vi "SeCrTs-DI SEQ MAIN.vi"(8 "error in":errorcluster, 11 "Message Queue":refnum<queue>) -> (0 "error Out":errorcluster)   [LabVIEW 2022 SP3]
uses:
  <vilib>/Platform/TimedLoop/XDataNode/timing_clust.ctl
  <vilib>/Platform/TimedLoop/XDataNode/nitl_modes.ctl
  <vilib>/Platform/TimedLoop/XDataNode/wakeup.ctl
  RT Controls/SeCrTs-FGV Read write.ctl
  <vilib>/platform/TimedLoop/XDataNode/XDataNode.xnode
  <vilib>/Platform/TimedLoop/XDataNode/XDNodeRunTimeDep.lvlib
panel:
  out "output array":string[](array[string])
  out "x-y":u32
  out "Numeric":i32
  out "Failure \ncase Seq":string[](array[string])
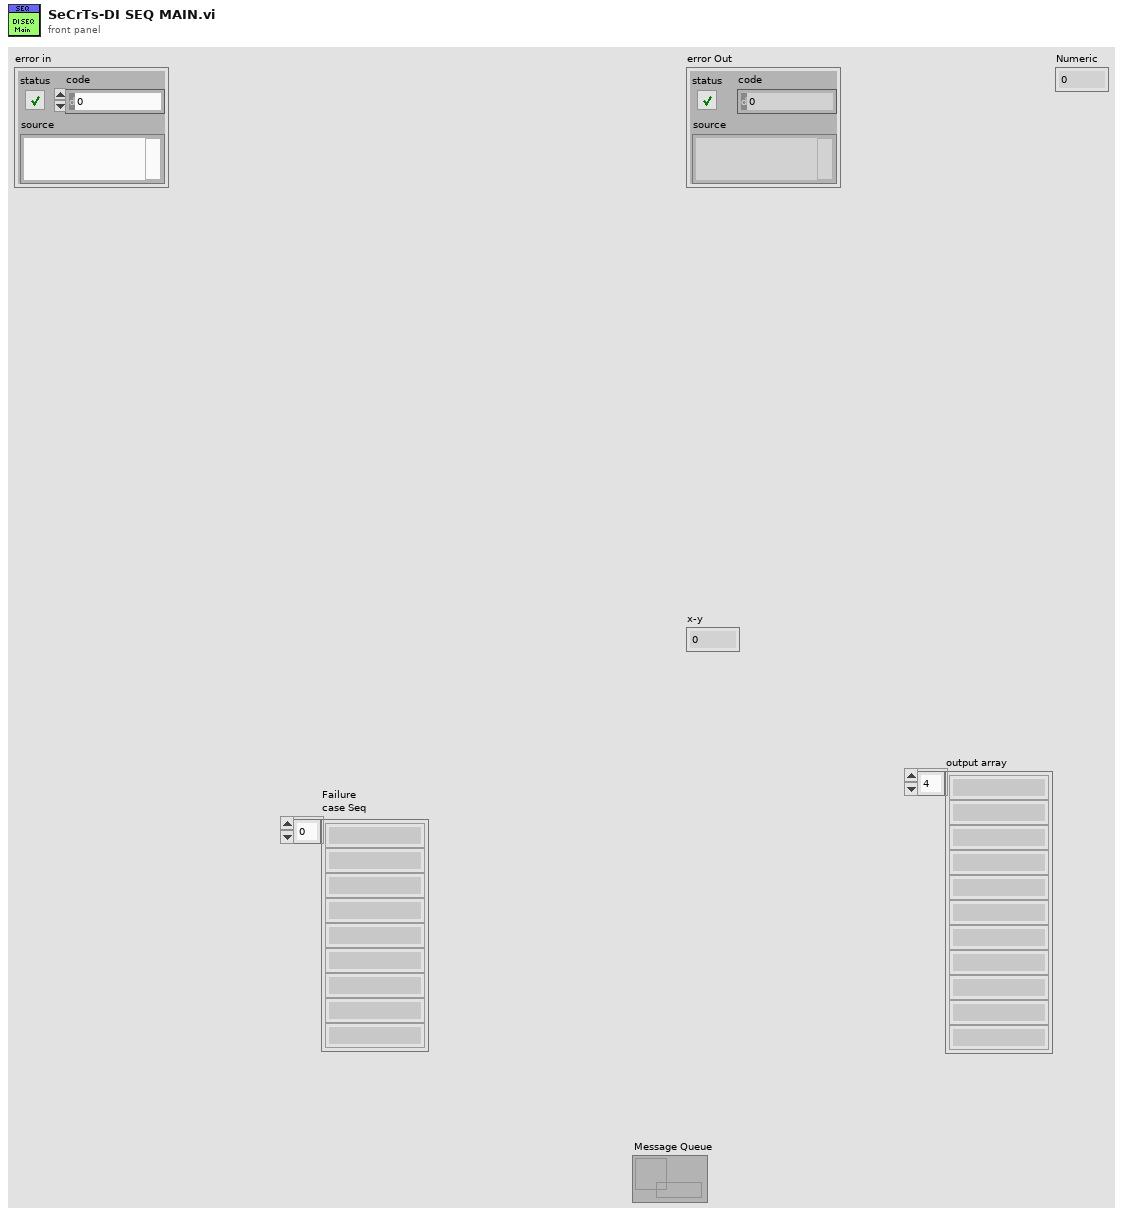
[diagram p1: front panel]
types:
  T1 = typedef "XDNodeRunTimeDep.lvlib/timing_clust.ctl" = cluster{"Expected End [f-1]":u64, "Actual End [f-1]":u64, "Finished Late? [f-1]":bool, "Expected End [i-1]":u64, "Actual End [i-1]":u64, "Finished Late? [i-1]":bool, "Expected Start [i]":u64, "Actual Start [i]":u64, "Expected Start [f]":u64, "Actual Start [f]":u64, "Source Name":string, "Structure Name":string, "Period":i64, "Deadline":i64, "Offset":i64, "Start":i64, "Priority":i32, "Timeout":i32, "Mode":T2, "Wakeup Reason":T3, "Error":errorcluster, "Source Type":string, "Secondary Source Type":string, "Global End Time":u64, "Global Start Time":u64, "Frame Duration":u64, "Iteration Duration":u64, "Assigned CPU":i32, "I/O Scan Engine Mode":u32}
  T2 = typedef "XDNodeRunTimeDep.lvlib/nitl_modes.ctl" = enum32{"No Change", "Process missed periods, maintain original phase", "Discard missed periods, maintain original phase", "Process missed periods, ignore original phase", "Discard missed periods, ignore original phase"}
  T3 = typedef "XDNodeRunTimeDep.lvlib/wakeup.ctl" = enum32{"Normal", "Aborted", "Asynchronous wakeup", "Timing source error", "Timed loop error", "Timeout"}
  T4 = typedef "SeCrTs-FGV Read write.ctl" = enum16{"Write", "Read"}
  T5 = cluster{"Start DAQ":bool, "Stop DAQ":bool, "RT Stop":bool, "RT Exit":bool, "Start Seq":bool}
  T6 = cluster{"Manual HOLD":bool, "Automatic Hold AI":bool, "Abort":bool, "Automatic Hold DI":bool}
  T7 = cluster{cluster{"Sr. No.":string, "Time CDT":string, "Component ID":string, "Data Type":string, "Condition":string, "Range/Position":string, "No of Samples for Pass":string, "Event Duration":string, "Continuous /Cumulative":string, "Expected Delay":string, "Failure case Seq":string, "Current Sequence":string}[]}[]
  T8 = cluster{"Sr. No.":string, "Time CDT":string, "Component ID":string, "Data Type":string, "Condition":string, "Range/Position":string, "No of Samples for Pass":string, "Event Duration":string, "Continuous /Cumulative":string, "Expected Delay":string, "Failure case Seq":string, "Current Sequence":string}[]
  T9 = cluster{"Sr. No.":string, "Time CDT":string, "Component ID":string, "Data Type":string, "Condition":string, "Range/Position":string, "No of Samples for Pass":string, "Event Duration":string, "Continuous /Cumulative":string, "Expected Delay":string, "Failure case Seq":string, "Current Sequence":string}
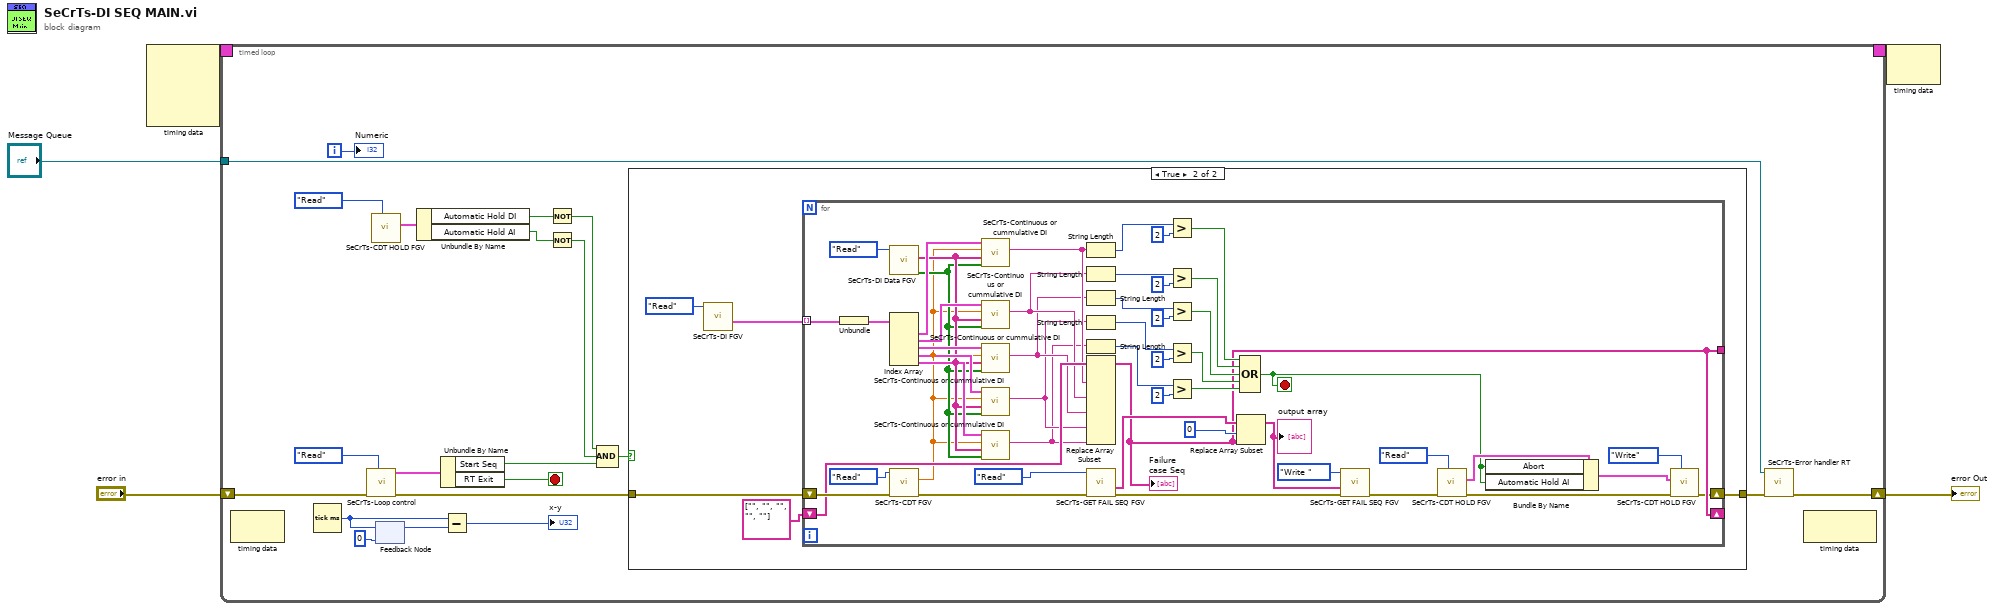
[diagram p0: block diagram]
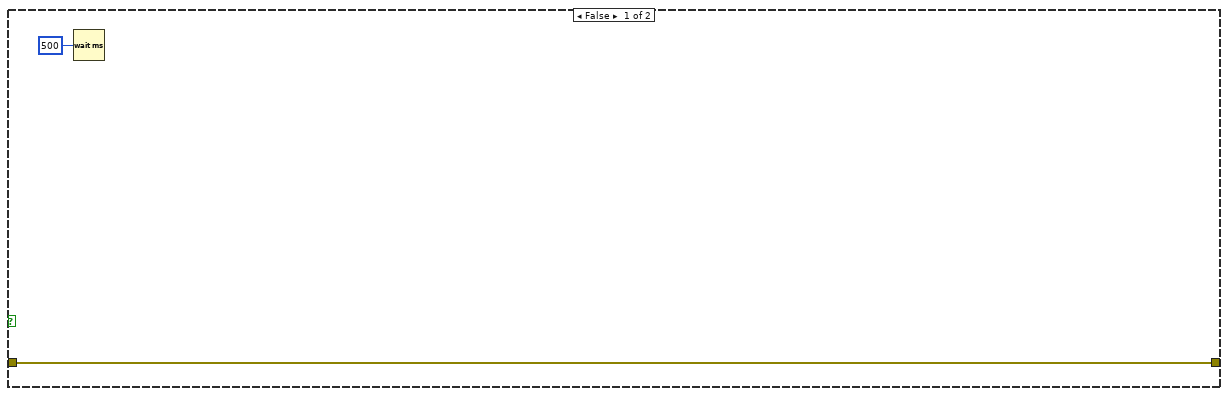
[diagram p2: hidden frame]
diagram:
  n1 = node-c288() -> (w3:T1)  [unwired: 4 in]
  n2 = timed-loop {
    shift-right: [w15] -> w5
    shift-left: "error in" -> [w19]
    timing: w3 -> [_]
    timing-out: [_] -> w2
    tunnel: "Message Queue" -> [w8]
    i -> [w26]
    stop <- w17 stop-if-true
    n3 = node-c288() -> ()  [unwired: 1 in, 1 out]
    n4 = Tick Count (ms)() -> (millisecond timer value=w24:u32)
    n5 = call "SeCrTs-Loop control.vi"("Action"=enum16{"Init", "Write", "Read"}."Read", "error in (no error)"=w19) -> ("error Out"=w18:errorcluster, "Loop Control out"=w20:T5)  [unwired: 8 in]
    n6 = call "SeCrTs-CDT HOLD FGV.vi"("Write/Read"=enum16{"Write", "Read"}."Read") -> ("HOLD and Abort Out"=w7:T6)  [unwired: 7 in, 1 out]
    n7 = feedback-in #1(w24) -> ()
    n8 = feedback #1(u32 0 ("millisecond timer value")) -> (w25:u32)
    n9 = Unbundle By Name(w7) -> ("Automatic Hold DI"=w10:bool, "Automatic Hold AI"=w12:bool)
    n10 = Unbundle By Name(w20) -> ("Start Seq"=w6:bool, "RT Exit"=w17:bool)
    n11 = Subtract(x=w24, y=w25) -> (x-y=→"x-y":u32)
    n12 = Not(x=w10) -> (.not. x?=w9:bool)
    n13 = Not(x=w12) -> (.not. x?=w13:bool)
    n14 = Compound Arithmetic op=AND(w9, w13, w6) -> (w11:bool)
    n15 = case shown="True" w11 {
      tunnel: w18 -> [w30 w35]
      tunnel: [w30 w31] -> w16
      frame False {
        n16 = Wait (ms)(milliseconds to wait=u32 500) -> ()  [unwired: 1 out]
      }
      frame True {
        n17 = call "SeCrTs-DI FGV.vi"("Enum"=enum16{"Read", "Write "}."Read") -> ("DI Seq  OUT"=w32:T7)  [unwired: 9 in, 1 out]
        n18 = for {
          tunnel: w32 -> [w79] mode=indexing
          shift-right: [w38] -> w31
          shift-left: w35 -> [w77]
          shift-right: [w44] -> _
          shift-left: string[] ["", "", "", "", ""] ("array") -> [w76]
          tunnel: [w44] -> _
          stop <- w36 stop-if-true
          n19 = Unbundle(w79) -> (w78:T8)
          n20 = call "SeCrTs-DI Data FGV.vi"("Write/Read"=SeCrTs-FGV_Read_write."Read") -> ("DI Y LP"=w73:bool[], "DI Signal List LP"=w74:string[])  [unwired: 8 in, 1 out]
          n21 = Index Array(array=w78) -> (element #1=w84:T9, element #2=w83:T9, element #3=w82:T9, element #4=w81:T9, element #5=w80:T9)  [unwired: 5 in]
          n22 = call "SeCrTs-CDT FGV.vi"("error in (no error)"=w77, "Write/Read"=enum16{"Write", "Read"}."Read") -> ("error Out"=w66:errorcluster, "CDT Out"=w67:dbl)  [unwired: 8 in]
          n23 = call "SeCrTs-Continuous or cummulative DI.vi"("DI   data"=w73, "DI Channels Name"=w74, "CDT"=w67, "output cluster"=w84) -> ("Failure case Seq"=w54:string)  [unwired: 6 in, 1 out]
          n24 = call "SeCrTs-Continuous or cummulative DI.vi"("DI   data"=w73, "DI Channels Name"=w74, "CDT"=w67, "output cluster"=w83) -> ("Failure case Seq"=w53:string)  [unwired: 6 in, 1 out]
          n25 = call "SeCrTs-Continuous or cummulative DI.vi"("DI   data"=w73, "DI Channels Name"=w74, "CDT"=w67, "output cluster"=w82) -> ("Failure case Seq"=w52:string)  [unwired: 6 in, 1 out]
          n26 = call "SeCrTs-Continuous or cummulative DI.vi"("DI   data"=w73, "DI Channels Name"=w74, "CDT"=w67, "output cluster"=w81) -> ("Failure case Seq"=w51:string)  [unwired: 6 in, 1 out]
          n27 = call "SeCrTs-Continuous or cummulative DI.vi"("DI   data"=w73, "DI Channels Name"=w74, "CDT"=w67, "output cluster"=w80) -> ("Failure case Seq"=w50:string)  [unwired: 6 in, 1 out]
          n28 = String Length(string=w54) -> (length=w59:i32)
          n29 = String Length(string=w53) -> (length=w58:i32)
          n30 = String Length(string=w52) -> (length=w57:i32)
          n31 = String Length(string=w51) -> (length=w56:i32)
          n32 = String Length(string=w50) -> (length=w55:i32)
          n33 = Replace Array Subset(array=w76, new element #1=w54, new element #2=w53, new element #3=w52, new element #4=w51, new element #5=w50) -> (w44:string[])  [unwired: 5 in]
          "Failure \ncase Seq" <- w44
          n34 = call "SeCrTs-GET FAIL SEQ FGV.vi"("error in"=w66, "Enum"=enum16{"Read", "Write "}."Read") -> ("error out"=w65:errorcluster, "Failure \ncase Seq"=w70:string[])  [unwired: 8 in]
          n35 = Greater?(x=w59, y=2) -> (0:w49:bool)
          n36 = Greater?(x=w58, y=2) -> (0:w48:bool)
          n37 = Greater?(x=w57, y=2) -> (0:w47:bool)
          n38 = Greater?(x=w56, y=2) -> (0:w46:bool)
          n39 = Greater?(x=w55, y=2) -> (0:w45:bool)
          n40 = Replace Array Subset(array=w70, new element=w44, index=0) -> (w68:string[])
          "output array" <- w68
          n41 = Compound Arithmetic op=OR(w49, w48, w47, w46, w45) -> (w36:bool)
          n42 = call "SeCrTs-GET FAIL SEQ FGV.vi"("error in"=w65, "Failure \ncase Seq"=w68, "Enum"=enum16{"Read", "Write "}."Write ") -> ("error out"=w37:errorcluster)  [unwired: 7 in, 1 out]
          n43 = call "SeCrTs-CDT HOLD FGV.vi"("Write/Read"=enum16{"Write", "Read"}."Read", "error in (no error)"=w37) -> ("error Out"=w41:errorcluster, "HOLD and Abort Out"=w40:T6)  [unwired: 6 in]
          n44 = Bundle By Name(cluster=w40, "Abort"=w36, "Automatic Hold AI"=w36) -> (w39:T6)
          n45 = call "SeCrTs-CDT HOLD FGV.vi"("Write/Read"=enum16{"Write", "Read"}."Write", "error in (no error)"=w41, "HOLD and Abort"=w39) -> ("error Out"=w38:errorcluster)  [unwired: 5 in, 1 out]
        }
      }
    }
    n46 = call "SeCrTs-Error handler RT.vi"("error in"=w16, "Message Queue"=w8) -> ("error out"=w15:errorcluster)  [unwired: 8 in, 1 out]
    n47 = node-c288() -> ()  [unwired: 1 in, 1 out]
    "Numeric" <- w26
  }
  "error Out" <- w5
  n48 = node-c288(w2) -> ()  [unwired: 1 out]
